vi "Launch_trial.vi"(7 "Trial sequence":cluster{"Sequence name":string, "Active":bool}[](array[cluster]), 11 "State in":T1) -> (0 "Remaining trials":cluster{"Sequence name":string, "Active":bool}[](array[cluster]), 3 "State out":T1)   [LabVIEW 2016]
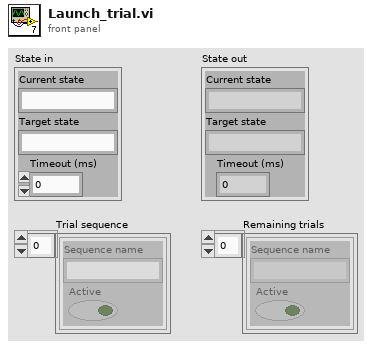
[diagram p1: front panel]
types:
  T1 = cluster{"Current state":string, "Target state":string, "Timeout (ms)":dbl}
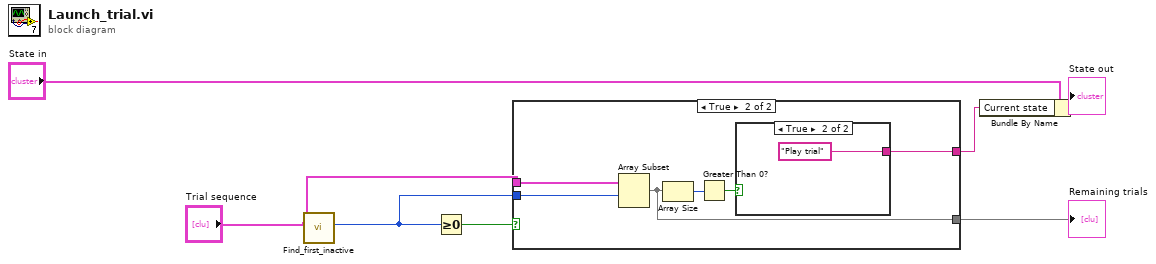
[diagram p0: block diagram]
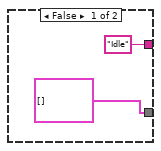
[diagram p2: hidden frame]
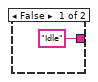
[diagram p3: hidden frame]
diagram:
  n1 = call "Find_first_inactive.vi"("Trial sequence"="Trial sequence") -> ("First inactive"=w5:i32)  [unwired: 10 in]
  n2 = Greater Or Equal To 0?(x=w5) -> (x >= 0?=w6:bool)
  n3 = case shown="True" w6 {
    tunnel: "Trial sequence" -> [_ w15]
    tunnel: [cluster{"Sequence name":string, "Active":bool}[] [] w14] -> w4
    tunnel: w5 -> [_ w13]
    tunnel: ["Idle" ("Current state") w10] -> w7
    frame False {
    }
    frame True {
      n4 = Array Subset(array=w15, index=w13) -> (w14:cluster{"Sequence name":string, "Active":bool}[])  [unwired: 1 in]
      n5 = Array Size(array=w14) -> (size(s)=w12:i32)
      n6 = Greater Than 0?(x=w12) -> (x > 0?=w11:bool)
      n7 = case shown="True" w11 {
        tunnel: ["Idle" ("Current state") "Play trial" ("Current state")] -> w10
        frame False {
        }
        frame True {
        }
      }
    }
  }
  "Remaining trials" <- w4
  n8 = Bundle By Name(cluster="State in", "Current state"=w7) -> (→"State out":T1)
